vi "DecisionMaker.vi"(0 "Trajectory Network":T2(array[cluster]), 1 "Change to state":i32, 2 "Vref":dbl, 3 "K":dbl, 4 "Platooning distances":dbl[](array[numeric]), 5 "Current State In":i32[](array[numeric]), 6 "Set MasterID":i32(ring) items=["None", "Blue Truck", "Black Truck", "Red Truck", "Grey Truck", "DarkGrey Truck"], 7 "Current WP In":i32[](array[numeric]), 8 "MyID":u8, 9 "Distance2Master":dbl[](array[numeric]), 11 "PlatoonArray":i32[](array[numeric]), 15 "Traffic Lights":T1, 16 "Trucks Poses":dbl[][](array[numeric]), 17 "d2TLFinal":dbl[](array[numeric])) -> (12 "d":dbl, 13 "dref":dbl, 20 "Current State Out":i32, 25 "VrefOut":dbl, 26 "CurrentWPOut":i32, 27 "Trajectory WP Out":dbl[][](array[numeric]))   [LabVIEW 2013]
uses:
  Global.vi
  <vilib>/imath/engines/lvmath2/RunTimeEngine/ErrorHandling/NIMS_Finalize Error.vi
  <vilib>/imath/engines/lvmath2/RunTimeEngine/BuiltInFunctions/size/NIMS_I32=size(GM,I32).vi
  <instcachedir>/0/NIMS_I32=size(GM,I32)_0501686D1A7F4581B546512A0CE6115B.lvgen/NIMS_I32=size(GM,I32)_0501686D1A7F4581B546512A0CE6115B_004.vi
  <vilib>/imath/engines/lvmath2/RunTimeEngine/BuiltInFunctions/zeros/NIMS_V=zeros(I32,I32).vi
  <vilib>/imath/engines/lvmath2/RunTimeEngine/ErrorHandling/NIMS_Create Error From Enums.vi
  <vilib>/imath/engines/lvmath2/RunTimeEngine/IndexRead/NIMS V(S).vi
  <instcachedir>/0/NIMS V(S)_0488751826AF41519A22953C041130DC.lvgen/NIMS V(S)_0488751826AF41519A22953C041130DC_002.vi
  <vilib>/imath/engines/lvmath2/RunTimeEngine/IndexReplace/NIMS V(S)=S.vi
  <instcachedir>/0/NIMS V(S)=S_66A18068148B4981A312229A93EA5C06.lvgen/NIMS V(S)=S_66A18068148B4981A312229A93EA5C06_004.vi
  <vilib>/imathl/engines/lvmath/Functions/Error Handling/Create Error.vi
  <vilib>/imath/engines/lvmath2/RunTimeEngine/NodeEndStatement/NIMS_NodeEndStatement_Output.vi
  <instcachedir>/0/NIMS_NodeEndStatement_Output_53EC0D466D134D7ABD903AC30B43404B.lvgen/NIMS_NodeEndStatement_Output_53EC0D466D134D7ABD903AC30B43404B_010.vi
  <instcachedir>/0/NIMS_NodeEndStatement_Output_53EC0D466D134D7ABD903AC30B43404B.lvgen/NIMS_NodeEndStatement_Output_53EC0D466D134D7ABD903AC30B43404B_004.vi
  <instcachedir>/0/NIMS_NodeEndStatement_Output_53EC0D466D134D7ABD903AC30B43404B.lvgen/NIMS_NodeEndStatement_Output_53EC0D466D134D7ABD903AC30B43404B_001.vi
  <vilib>/imath/engines/lvmath/Functions/Error Handling/MergeErrorsWrapper.vi
  <vilib>/imath/engines/lvmath2/RunTimeEngine/IndexRead/NIMS M(S,S).vi
  <instcachedir>/0/NIMS M(S,S)_AC51E74150A542F7991B9634C66F3096.lvgen/NIMS M(S,S)_AC51E74150A542F7991B9634C66F3096_000.vi
  <vilib>/imath/engines/lvmath2/RunTimeEngine/BuiltInFunctions/deg_to_rad/NIMS_deg_to_rad.vi
  <instcachedir>/0/NIMS_deg_to_rad_4A81D684CE8D4DD79924F5AB74D756E1.lvgen/NIMS_deg_to_rad_4A81D684CE8D4DD79924F5AB74D756E1_001.vi
  <vilib>/imath/engines/lvmath2/RunTimeEngine/BuiltInFunctions/atan2/NIMS_atan2.vi
  <instcachedir>/0/NIMS_atan2_A91AA4A7D42247EDBE8F76DB99AF04A4.lvgen/NIMS_atan2_A91AA4A7D42247EDBE8F76DB99AF04A4_000.vi
  <instcachedir>/0/NIMS V(S)_0488751826AF41519A22953C041130DC.lvgen/NIMS V(S)_0488751826AF41519A22953C041130DC_000.vi
  <vilib>/imath/engines/lvmath2/RunTimeEngine/BuiltInFunctions/length/NIMS_length(GM).vi
  <instcachedir>/0/NIMS_length(GM)_47CEC356FCE0482D9BA47DC61C99F2C7.lvgen/NIMS_length(GM)_47CEC356FCE0482D9BA47DC61C99F2C7_000.vi
  <vilib>/imath/engines/lvmath2/RunTimeEngine/BuiltInFunctions/rem/NIMS_rem_no checks.vi
  <instcachedir>/0/NIMS_rem_no checks_7935C26835844EFC868069820ED089DA.lvgen/NIMS_rem_no checks_7935C26835844EFC868069820ED089DA_008.vi
  <instcachedir>/0/NIMS V(S)_0488751826AF41519A22953C041130DC.lvgen/NIMS V(S)_0488751826AF41519A22953C041130DC_004.vi
  <instcachedir>/0/NIMS M(S,S)_AC51E74150A542F7991B9634C66F3096.lvgen/NIMS M(S,S)_AC51E74150A542F7991B9634C66F3096_003.vi
  <vilib>/imath/engines/lvmath2/RunTimeEngine/IndexRead/NIMS M(S,$).vi
  <instcachedir>/0/NIMS M(S,$)_F24F360562DE41D8BE234322A2E15C65.lvgen/NIMS M(S,$)_F24F360562DE41D8BE234322A2E15C65_000.vi
  <vilib>/imath/engines/lvmath2/RunTimeEngine/BuiltInFunctions/is_nan/NIMS_is_nan.vi
  <instcachedir>/0/NIMS_is_nan_BCCD798162CC49E3A8E57072444F6EB6.lvgen/NIMS_is_nan_BCCD798162CC49E3A8E57072444F6EB6_003.vi
  <vilib>/imath/engines/lvmath2/RunTimeEngine/BuiltInFunctions/sum/NIMS_sum(GV).vi
  <instcachedir>/0/NIMS_sum(GV)_67F5EC36BC034E54A6BEC5B0673C00E5.lvgen/NIMS_sum(GV)_67F5EC36BC034E54A6BEC5B0673C00E5_000.vi
panel:
  in  "Transition WP":i32[][](array[numeric])=[[-1, -1, -1, -1], [-1, -1, -1, -1], [-1, -1, 5, 1], [-1, -1, 50, 25]]
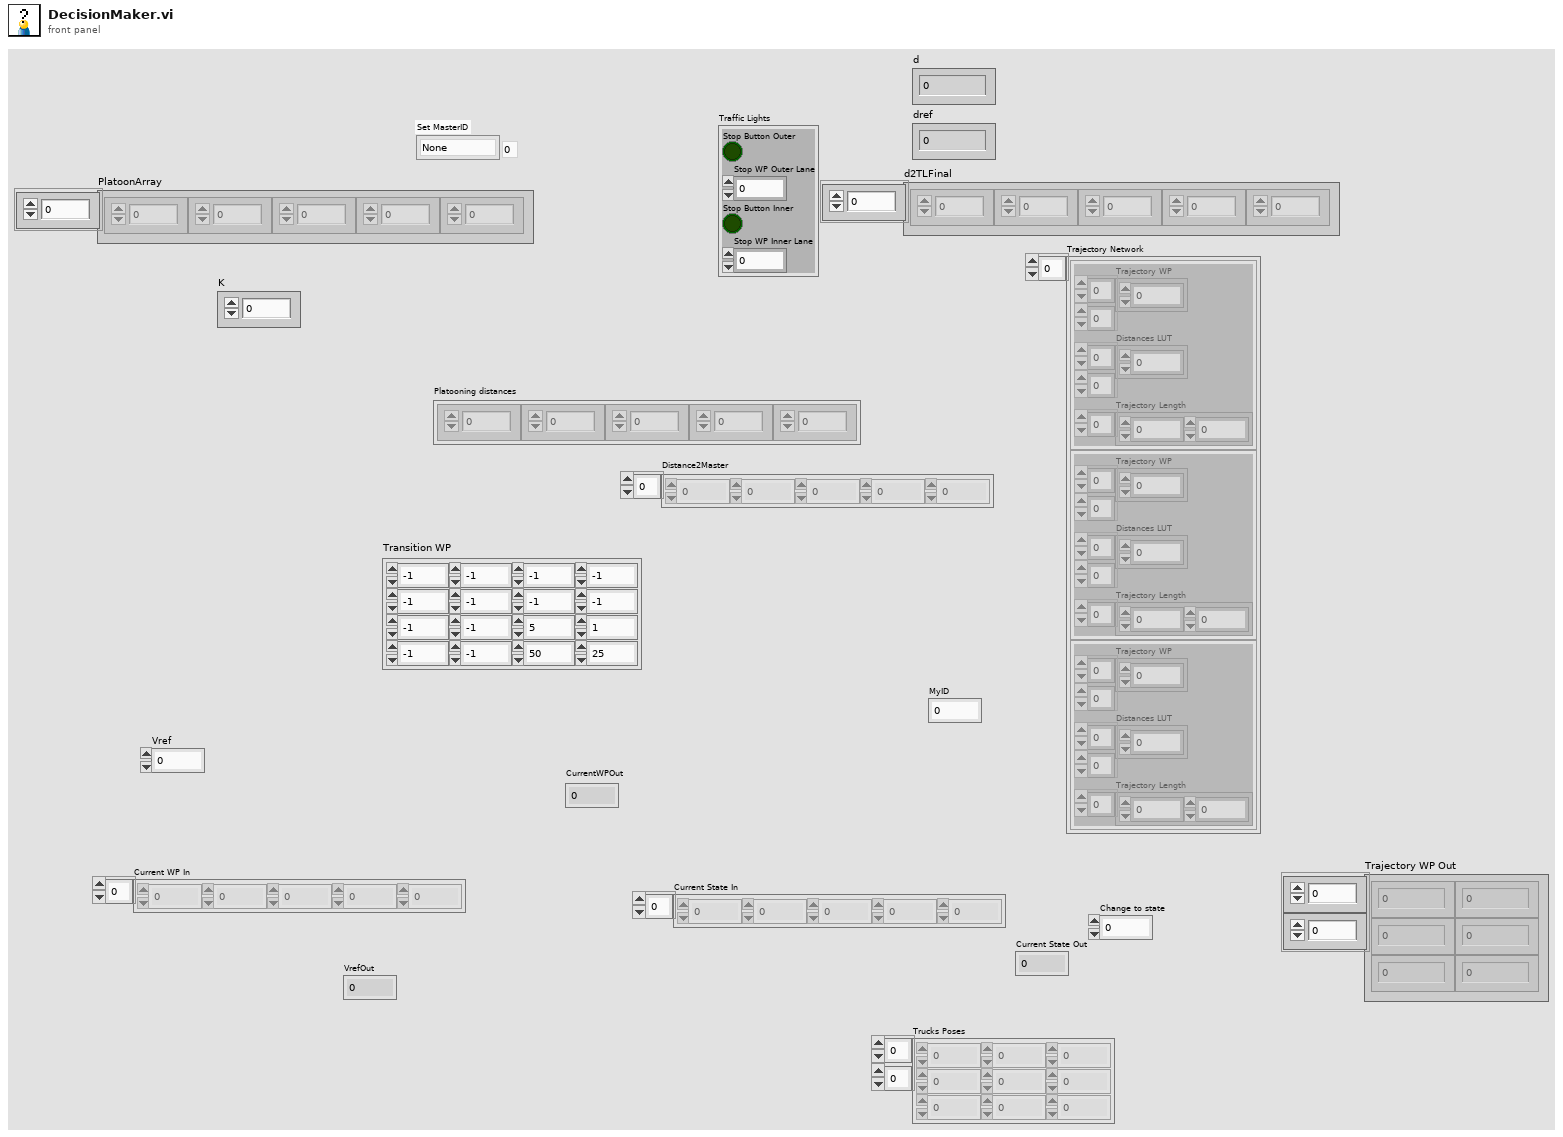
[diagram p1: front panel]
types:
  T1 = cluster{"Stop Button Outer":bool, "Stop WP Outer Lane":i32, "Stop Button Inner":bool, "Stop WP Inner Lane ":i32}
  T2 = cluster{"Trajectory WP":dbl[][], "Distances LUT":dbl[][], "Trajectory Length":i32[]}[]
  T3 = cluster{"Trajectory WP":dbl[][], "Distances LUT":dbl[][], "Trajectory Length":i32[]}
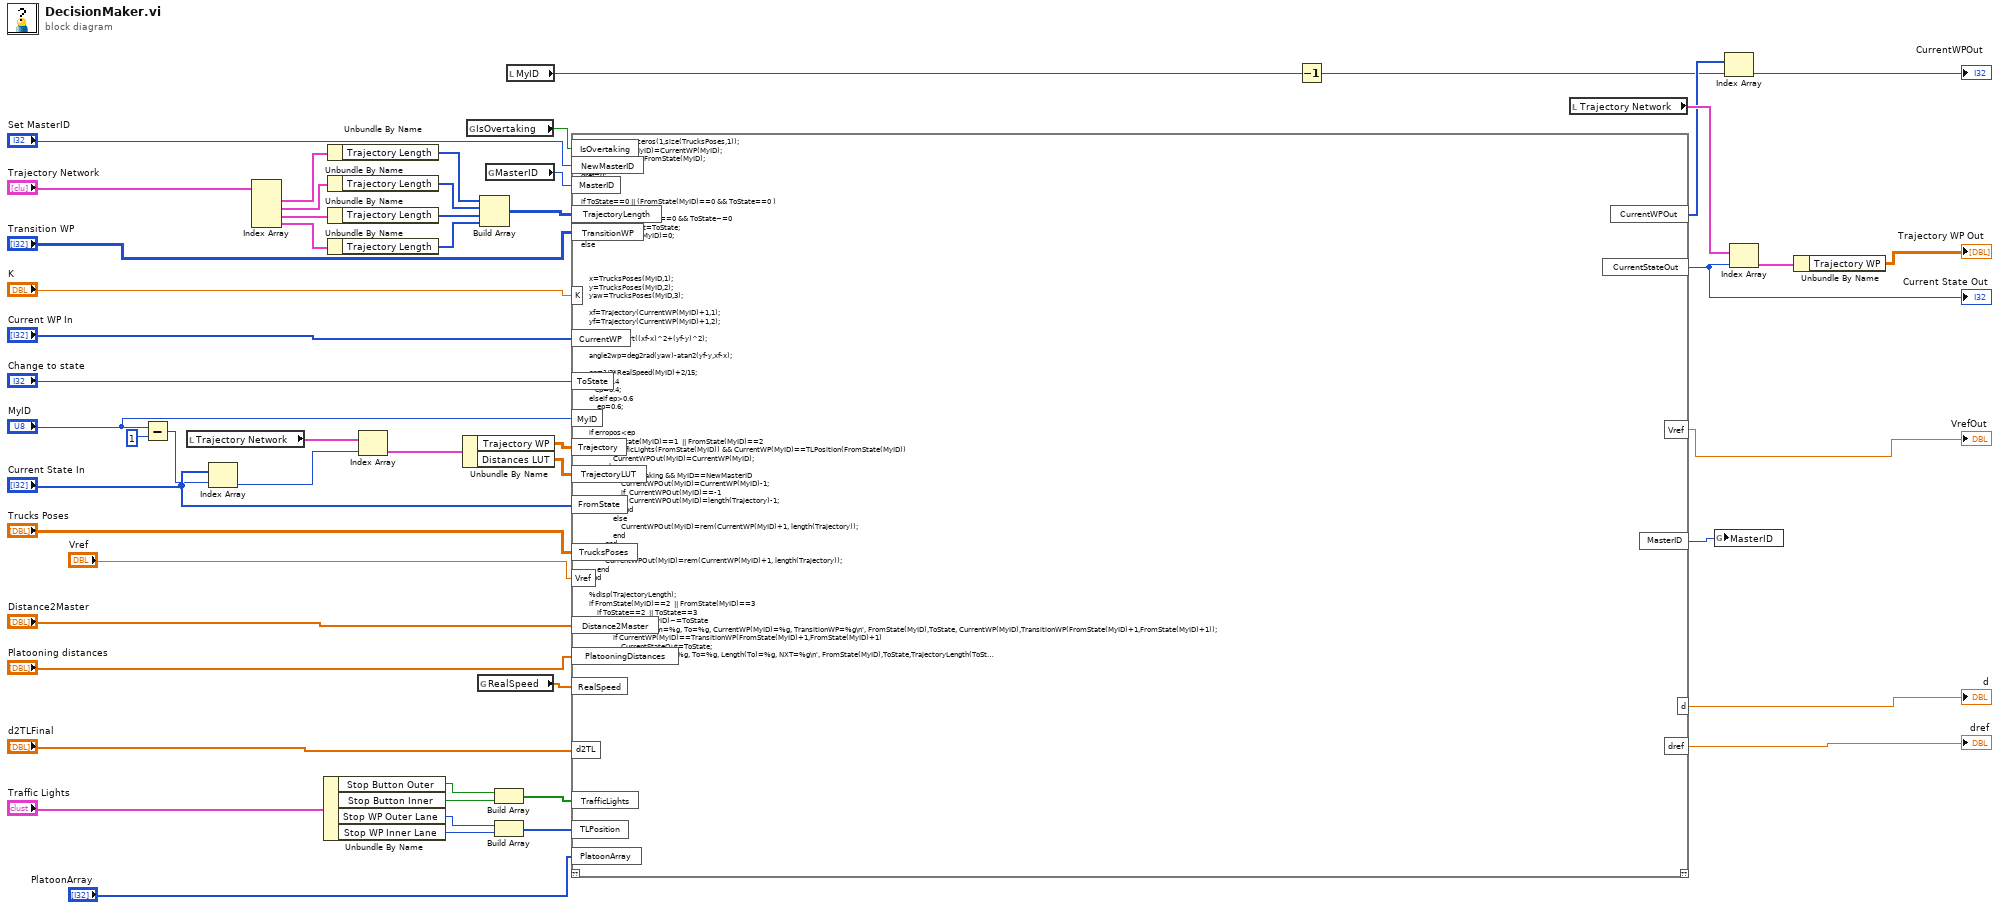
[diagram p0: block diagram]
diagram:
  n1 = Subtract(x="MyID", y=u8 1) -> (x-y=w28:u8)
  n2 = local read "Trajectory Network"() -> (w40:T2)
  n3 = Index Array(array="Current State In", index=w28) -> (element=w32:i32)
  n4 = Index Array(array="Trajectory Network") -> (element #1=w44:T3, element #2=w42:T3, element #3=w43:T3, element #4=w37:T3)  [unwired: 4 in]
  n5 = Unbundle By Name("Traffic Lights") -> ("Stop Button Outer"=w26:bool, "Stop Button Inner"=w25:bool, "Stop WP Outer Lane"=w23:i32, "Stop WP Inner Lane"=w24:i32)
  n6 = Unbundle By Name(w44) -> ("Trajectory Length"=w51:i32[])
  n7 = Unbundle By Name(w42) -> ("Trajectory Length"=w50:i32[])
  n8 = Unbundle By Name(w43) -> ("Trajectory Length"=w49:i32[])
  n9 = Unbundle By Name(w37) -> ("Trajectory Length"=w36:i32[])
  n10 = Index Array(array=w40, index=w32) -> (element=w39:T3)
  n11 = Unbundle By Name(w39) -> ("Trajectory WP"=w20:dbl[][], "Distances LUT"=w19:dbl[][])
  n12 = global read "Global.vi" "IsOvertaking"() -> (w14:bool)
  n13 = global read "Global.vi" "RealSpeed"() -> (w33:dbl[])
  n14 = Build Array(w51, w50, w49, w36) -> (w5:i32[][])
  n15 = global read "Global.vi" "MasterID"() -> (w4:i32)
  n16 = Build Array(w26, w25) -> (w22:bool[])
  n17 = Build Array(w23, w24) -> (w21:i32[])
  n18 = local read "MyID"() -> (w12:u8)
  n19 = mathscript code="CurrentWPOut=zeros(1,size(TrucksPoses,1));\nCurrentWPOut(MyID)=CurrentWP(MyID);\nCurrentStateOut=FromState(MyID);\nd=0;\ndref=0;\n\n\nif ToState==0 || (FromState(MyID)==0 && ToState==0 )\n    CurrentStateOut=0;\nelseif FromState(MyID)==0 && ToState~=0\n    CurrentStateOut=ToState;\n    CurrentWPOut(MyID)=0;\nelse\n    \n    \n    \n    x=TrucksPoses(MyID,1);\n    y=TrucksPoses(MyID,2);\n    yaw=TrucksPoses(MyID,3);\n    \n    xf=Trajectory(CurrentWP(MyID)+1,1);\n    yf=Trajectory(CurrentWP(MyID)+1,2);\n    \n    erropos=sqrt((xf-x)^2+(yf-y)^2);\n    \n    angle2wp=deg2rad(yaw)-atan2(yf-y,xf-x);\n    \n    ep=1/3*RealSpeed(MyID)+2/15;\n    if ep<0.4\n       ep=0.4;\n    elseif ep>0.6\n        ep=0.6;\n    end\n\n    if erropos<ep\n        if FromState(MyID)==1  || FromState(MyID)==2\n            if  TrafficLights(FromState(MyID)) && CurrentWP(MyID)==TLPosition(FromState(MyID))\n                CurrentWPOut(MyID)=CurrentWP(MyID);\n            else\n                if IsOvertaking && MyID==NewMasterID\n                    CurrentWPOut(MyID)=CurrentWP(MyID)-1;\n                    if  CurrentWPOut(MyID)==-1\n                        CurrentWPOut(MyID)=length(Trajectory)-1;\n                    end\n                else\n                    CurrentWPOut(MyID)=rem(CurrentWP(MyID)+1, length(Trajectory));\n                end\n            end\n        else\n            CurrentWPOut(MyID)=rem(CurrentWP(MyID)+1, length(Trajectory));\n        end\n    end\n    \n    %disp(TrajectoryLength);\n    if FromState(MyID)==2  || FromState(MyID)==3\n        if ToState==2  || ToState==3\n            if FromState(MyID)~=ToState\n                %fprintf('From=%g, To=%g, CurrentWP(MyID)=%g, TransitionWP=%g\\n', FromState(MyID),ToState, CurrentWP(MyID),TransitionWP(FromState(MyID)+1,FromState(MyID)+1));\n                if CurrentWP(MyID)==TransitionWP(FromState(MyID)+1,FromState(MyID)+1)\n                    CurrentStateOut=ToState;\n                    %fprintf('From=%g, To=%g, Length(To)=%g, NXT=%g\\n', FromState(MyID),ToState,TrajectoryLength(ToState+1,1),TransitionWP(FromState(MyID)+1,FromState(MyID)+1)+1);\n                    CurrentWPOut(MyID)=TransitionWP(FromState(MyID)+1,ToState+1);\n                    if MyID==MasterID\n                        MasterID=0;\n                    end\n                end\n            end\n        end\n    end\n    \n    if MyID==NewMasterID && IsOvertaking\n        if MasterID~=0\n            Vref=K*RealSpeed(MasterID);\n        else\n            Vref=RealSpeed(MyID);\n        end\n    end\n    \n    D=10*Vref;\n    \n    if MasterID~=MyID && MasterID~=0 && FromState(MyID)==FromState(MasterID)\n        dref=PlatooningDistances(MasterID);\n        d=Distance2Master(MyID);\n        if RealSpeed(MasterID)>0.1\n            %Vref=RealSpeed(MasterID)+(d-dref)^3;\n            Vref=RealSpeed(MasterID)*d/dref;\n            %Vref=RealSpeed(MasterID)*d/(2*dref) + RealSpeed(MasterID)/2;\n            if Vref>K*RealSpeed(MasterID)\n                Vref=K*RealSpeed(MasterID);\n            elseif Vref<0\n                Vref=0;\n                totalerror_v_previous=0;\n            end\n        elseif d<=dref+0.2 || sum(is_nan(TrucksPoses(MasterID,:)))>0\n            Vref=0;\n        elseif d<=D*dref\n            %Vref=(d-dref)*Vref/((D-1)*dref)+0.2;\n            Vref=(Vref-0.1)/(D*dref)*d+0.1;\n        end\n        \n    end\n    \n    dref2TL=0.3;\n    \n    if FromState(MyID)==1  || FromState(MyID)==2\n        if TrafficLights(FromState(MyID))\n            %    if MyID==MasterID || MasterID==0\n            if d2TL(MyID)<=dref2TL+0.2\n                Vref=0;\n            elseif d2TL(MyID)<=D*dref2TL\n                Vref=(Vref-0.1)/(D*dref2TL)*d2TL(MyID)+0.1;\n            end\n            %     end\n        end\n    end\n    \nend"("TransitionWP"="Transition WP", "FromState"="Current State In", "CurrentWP"="Current WP In", "ToState"="Change to state", "TrajectoryLength"=w5, "TrucksPoses"="Trucks Poses", "MyID"="MyID", "Trajectory"=w20, "MasterID"=w4, "Distance2Master"="Distance2Master", "PlatooningDistances"="Platooning distances", "RealSpeed"=w33, "Vref"="Vref", "TrafficLights"=w22, "TLPosition"=w21, "TrajectoryLUT"=w19, "d2TL"="d2TLFinal", "K"="K", "IsOvertaking"=w14, "NewMasterID"="Set MasterID", "PlatoonArray"="PlatoonArray") -> ("CurrentStateOut"=w45:i32, "CurrentWPOut"=w11:i32[], "MasterID"=w38:i32, "Vref"=→"VrefOut":dbl, "d"=→"d":dbl, "dref"=→"dref":dbl)  [unwired: 1 in, 1 out]
  "Current State Out" <- w45
  n20 = Decrement(x=w12) -> (x-1=w9:u8)
  n21 = local read "Trajectory Network"() -> (w17:T2)
  n22 = global write "Global.vi" "MasterID"(w38) -> ()
  n23 = Index Array(array=w11, index=w9) -> (element=→"CurrentWPOut":i32)
  n24 = Index Array(array=w17, index=w45) -> (element=w47:T3)
  n25 = Unbundle By Name(w47) -> ("Trajectory WP"=→"Trajectory WP Out":dbl[][])
